vi "GetOutputCount.vi"(8 "error in (no error)":errorcluster, 11 "session id in":i32) -> (0 "error out":errorcluster, 2 "OutputCount":i32, 3 "session id out":i32)   [LabVIEW 2017, in "libonnx_wrapper.lvlib"]
doc: "/**\n * @brief Получить количество выходов модели\n * \n * Возвращает число выходных тензоров, которые производит модель.\n * Модели классификации обычно имеют 1 выход, детекции объектов — несколько.\n * \n * @param sessionId [IN] ID сессии\n * \n * @return int32: Количество выходов (0 или больше)\n * @return int32: 0 если сессия не найдена или не загружена\n */\nint GetOutputCount(int sessionId);"
uses:
  libonnx_wrapper.lvlib
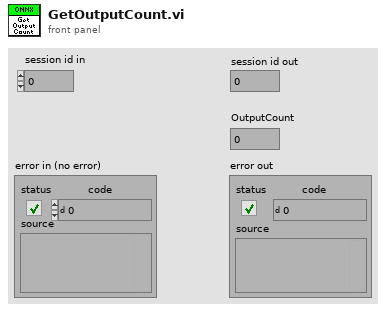
[diagram p1: front panel]
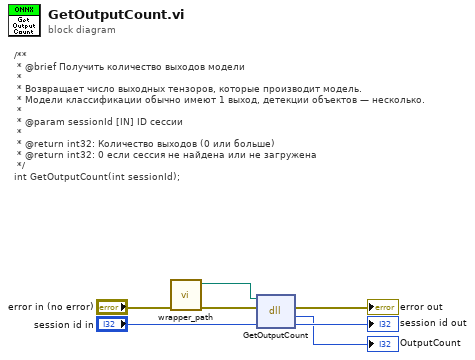
[diagram p0: block diagram]
diagram:
  # "/**\n * @brief Получить количество выходов модели\n * \n * Возвращает число выходных тензоров, которые производит модель.\n * Модели классификации обычно имеют 1 выход, детекции объектов — несколько.\n * \n * @param sessionId [IN] ID сессии\n * \n * @return int32: Количество выходов (0 или больше)\n * @return int32: 0 если сессия не найдена или не загружена\n */\nint GetOutputCount(int sessionId);"
  n1 = call "wrapper_path.vi"("error in (no error)"="error in (no error)") -> ("error out"=w5:errorcluster, "wrapper path"=w4:path)  [unwired: 9 in]
  n2 = dll-call lib="home/ivan/LabVIEWData/ONNX/Test/libonnx_wrapper/unix64/libonnx_wrapper.so" fn="GetOutputCount"(path in=w4, error in=w5, "sessionId"="session id in") -> (error out=→"error out":errorcluster, "OutputCount"=→"OutputCount":i32, "sessionId"=→"session id out":i32)  [unwired: 1 in, 1 out]
